vi "manipulate3Columns.vi"(8 "Col2Mul":dbl=1.0, 9 "Col1Mul":dbl=1.0, 10 "Col0Mul":dbl=1.0, 11 "Real Matrix":T1=[[2354.0, 1.0], [34.0, 3.0], [2354.0, 4.0], [34.0, 5.0], [235235.0, 2.0], [4545.0, 3.0], [34.0, 33.0], [23.0, 3.0], [235.0, 3.0]]) -> (3 "submatrix":T1)   [LabVIEW 2011]
uses:
  <vilib>/Analysis/Matrix/Datatypes/RealMatrix.ctl
  <vilib>/Analysis/Matrix/Numeric/Multiply/Multiply - RM,R.vi
  <vilib>/Analysis/Matrix/NI_Matrix.lvlib
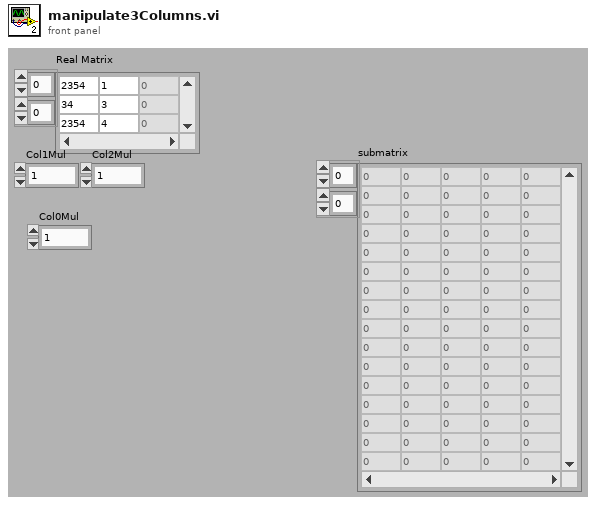
[diagram p1: front panel]
types:
  T1 = typedef "NI_Matrix.lvlib/RealMatrix.ctl" = dbl[][]
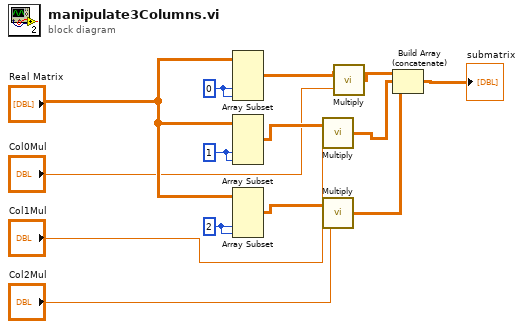
[diagram p0: block diagram]
diagram:
  w10 = 2 ("column 1")
  w13 = 1 ("column 1")
  w12 = 0 ("column 1")
  n1 = Array Subset(array="Real Matrix", index (col)=w12, length (col)=w12) -> (w7:T1)  [unwired: 2 in]
  n2 = Array Subset(array="Real Matrix", index (col)=w13, length (col)=w13) -> (w9:T1)  [unwired: 2 in]
  n3 = Array Subset(array="Real Matrix", index (col)=w10, length (col)=w10) -> (w5:T1)  [unwired: 2 in]
  n4 = call-poly <vilib>:"Multiply.vi"("Real Scalar c"="Col1Mul", "Real Matrix A"=w9) -> ("A * c"=w8:T1)
  n5 = call-poly <vilib>:"Multiply.vi"("Real Scalar c"="Col2Mul", "Real Matrix A"=w5) -> ("A * c"=w4:T1)
  n6 = call-poly <vilib>:"Multiply.vi"("Real Scalar c"="Col0Mul", "Real Matrix A"=w7) -> ("A * c"=w6:T1)
  n7 = Build Array (concatenate)(w6, w8, w4) -> (→"submatrix":T1)
